vi "Initialize MM Network.vi"(7 "Net Adress":string, 8 "error in (no error)":errorcluster, 11 "Sensor Engine Datas in":T1[](array[typedef])) -> (0 "error out":errorcluster, 3 "Sensor Engine Datas out":T1[](array[typedef]))   [LabVIEW 2023, in "MM.lvlib"]
uses:
  MM.lvlib
  Sensor Engine Data.ctl
  DataContainer/DataContainer.lvclass
  Shared/Protocol.ctl
  Shared/Vires VTD Shared.lvlib
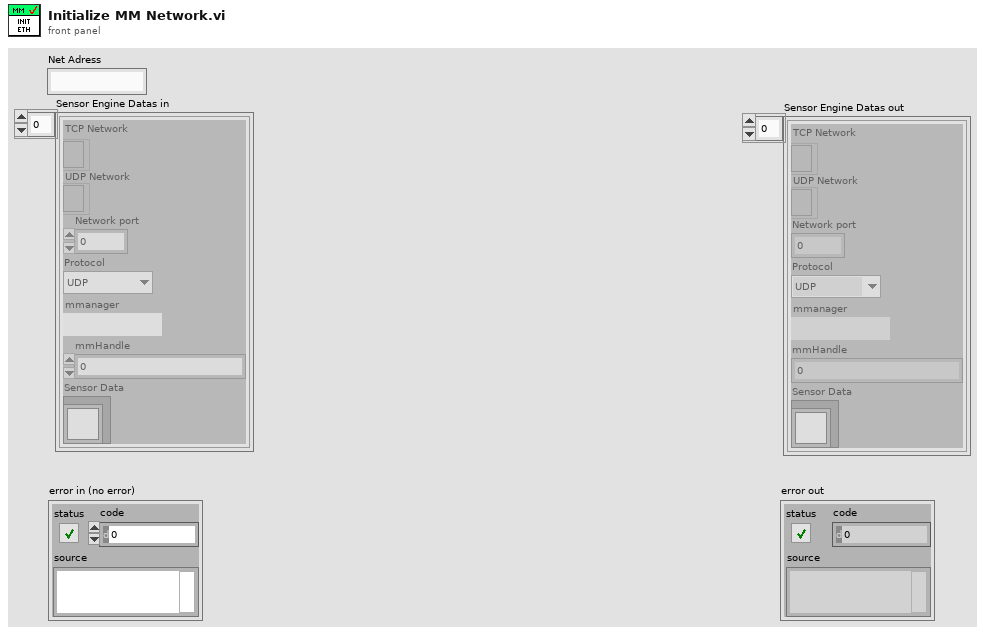
[diagram p1: front panel]
types:
  T1 = typedef "MM.lvlib/Sensor Engine Data.ctl" = cluster{"TCP Network":refnum<k5>, "UDP Network":refnum<k16>, "Network port":i32, "Protocol":T2, "mmanager":path, "mmHandle":u64, "Sensor Data":refnum<class "DataContainer.lvclass">}
  T2 = typedef "Vires VTD Shared.lvlib/Protocol.ctl" = enum16{"UDP", "TCP"}
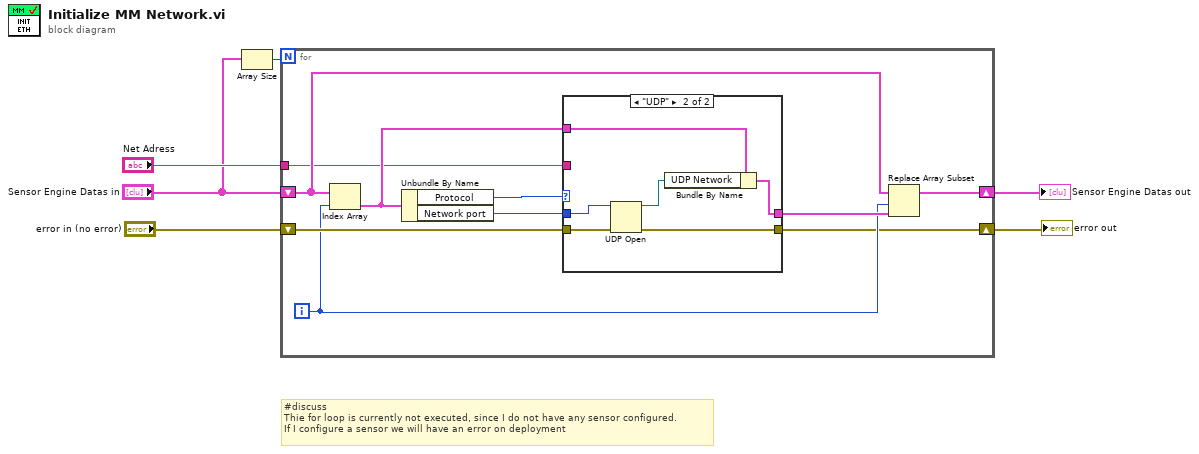
[diagram p0: block diagram]
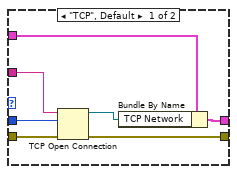
[diagram p2: hidden frame]
diagram:
  # "#discuss\nThie for loop is currently not executed, since I do not have any sensor configured.\nIf I configure a sensor we will have an error on deployment"
  n1 = Array Size(array="Sensor Engine Datas in") -> (size(s)=w2:i32)
  n2 = for {
    N: w2 -> [_]
    tunnel: "Net Adress" -> [w9]
    shift-right: [w7] -> w4
    shift-left: "error in (no error)" -> [w16]
    shift-right: [w14] -> w3
    shift-left: "Sensor Engine Datas in" -> [w15]
    i -> [w11]
    n3 = Index Array(array=w15, index=w11) -> (element=w13:T1)
    n4 = Unbundle By Name(w13) -> ("Protocol"=w10:T2, "Network port"=w8:i32)
    n5 = case shown="\"UDP\"" w10 {
      tunnel: w9 -> [w23 _]
      tunnel: w8 -> [w22 w24]
      tunnel: w16 -> [w21 w29]
      tunnel: [w20 w28] -> w7
      tunnel: w13 -> [w18 w27]
      tunnel: [w17 w26] -> w12
      frame "TCP", Default {
        n6 = TCP Open Connection(address=w23, remote port or service name=w22, error in (no error)=w21) -> (connection ID=w19:refnum<k5>, error out=w20:errorcluster)  [unwired: 2 in]
        n7 = Bundle By Name(cluster=w18, "TCP Network"=w19) -> (w17:T1)
      }
      frame "UDP" {
        n8 = UDP Open(8:w29, 11:w24) -> (port=w25:refnum<k16>, 0:w28:errorcluster)  [unwired: 3 in, 1 out]
        n9 = Bundle By Name(cluster=w27, "UDP Network"=w25) -> (w26:T1)
      }
    }
    n10 = Replace Array Subset(array=w15, new element=w12, index=w11) -> (w14:T1[])
  }
  "error out" <- w4
  "Sensor Engine Datas out" <- w3
